vi "LINX VI API Version.vi"() -> (1 "SubMinor":u8, 2 "Minor":u8, 3 "Major":u8=2)   [LabVIEW 2020, in "Device.lvlib"]
uses:
  Device.lvlib
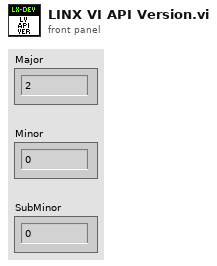
[diagram p1: front panel]
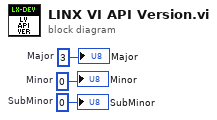
[diagram p0: block diagram]
diagram:
  w3 = u8 0  # SubMinor
  w2 = u8 0  # Minor
  w1 = u8 3  # Major
  "SubMinor" <- w3
  "Minor" <- w2
  "Major" <- w1
